vi "MarkedRobotStriker2.vi"(6 "atacando ao contrário?":bool=TRUE, 8 "Função":T1, 9 "id":u32, 10 "IA State Input":T3={"our_robots"=[], "enemy_robots"=[], "balls"=[], "geometry"={"line_width"=0, "field_length"=0, "field_width"=0, "boundary_width"=0, "referee_width"=0, "goal_width"=0, "goal_depth"=0, "goal_wall_width"=0, "center_circle_radius"=0, "defense_radius"=0, "defense_stretch"=0, "free_kick_from_defense_dist"=0, "penalty_spot_from_field_line_dist"=0, "penalty_line_from_spot_dist"=0}, "IA Judge"={"stage"="", "command"="", "our_goalie_id"=0.0, "enemy_goalie_id"=0.0, "command enum"=enum."Halt", "Time"=enum."Azul"}, "Received Timestamp"=timestamp(0 s since 1904-01-01), "Events"={"Touch"=FALSE, "Ball out"=FALSE, "id touch"=0.0, "Ball out of \nVision"=FALSE, "Ball inside \nGoalie area"=FALSE, "Robot not responding"=FALSE, "Robots responding status"=[1.0, 1.0, 1.0, 1.0, 1.0, 1.0], "Enemy Ball \nPossession"=FALSE, "Pass State"=FALSE, "id end of pass"=0.0, "Kick"=FALSE, "Id ini Possession"=0.0, "Ball Possesion"=FALSE, "Id Possesion"=0.0, "Direct Kick"=FALSE, "2nd Strk Ativo"=FALSE}}, 11 "AI Parameters":T2={"GotoKick"={"Dist do cone a frente"=150.0, "attacker farback"=1500.0, "Perto"=300.0, "min dist to kick"=150.0, "kick eps"=0.0, "Time to transition"=0.05}, "Attacker"={"CC chute"=0.09, "CC passe"=0.045, "Kick Force"=100.0, "ball-robot Kick"=200.0, "ball-robot Pass"=0.3, "drible\nAttk"=FALSE}, "Defender"={"D max"=1700.0, "Vel p/ robô av"=1000.0, "Kick Force"=100.0, "D atk-def"=0.0, "D farback"=0.0, "drible\ndef"=FALSE, "drible\ngoalie"=FALSE}, "Timeout"={"Field/v in x"=6.0, "Dist Robots"=300, "Dist up in y"=300}, "Pose Striker"={"dist"=200.0, "Numeric"=-4.0, "dist 2"=200.0, "drible\nstriker"=FALSE}, "Dist Stop"=300.0, "D ball out"=200, "D central gap "=150.0, "T pass"=0.0, "Force ++"=0.0, "range kick"=0.0, "Chute alto"=TRUE, "Marcador novo"=TRUE, "drible"=FALSE, "D drible"=300.0, "Versão Striker"=enum."3", "Defesa"=enum."ManMark", "Marcador"=enum."Marcar Segndo mais perigoso", "Receptor passe"=enum."2nd Striker", "Área"=enum."Quadrada"} {"D drible" format="%#_13g"; "D central gap" format="%#_13g"; "Dist Stop" format="%#_13g"; "Pose Striker"."Numeric" format="%#_13g"; "Defender"."Kick Force" format="%#_13g"; "Defender"."Vel p/ robô av" format="%#_13g"; "Attacker"."ball-robot Kick" format="%#_13g"; "Attacker"."Kick Force" format="%#_13g"; "Attacker"."CC passe" format="%#_13g"; "Attacker"."CC chute" format="%#_13g"; "GotoKick"."kick eps" format="%#_13g"; "GotoKick"."min dist to kick" format="%#_13g"; "GotoKick"."Perto" format="%#_13g"; "GotoKick"."attacker farback" format="%#_13g"; "GotoKick"."Dist do cone a frente" format="%#_13g"}) -> (2 "Dif. tempo\ninimigo bola":dbl, 3 "Robô marcado?":bool=TRUE, 7 "menor dist":dbl)   [LabVIEW 2017]
uses:
  Core/AI Input.ctl
  Core/AI Robot.ctl
  Functions Enum.ctl
  AttackerStates.ctl
  Path Planning/RRT/PathDests.ctl
  Path Planning/RRT/PathDest.ctl
  Core/AI Ball.ctl
  Core/Field Size.ctl
  Core/AI Judge.ctl
  Command Enum.ctl
  Util/Events/Events.ctl
  AI Parameters.ctl
  d3ae8bea-2540-4cab-b848-3da8b8f91e54.vi
  <vilib>/Array/Sort 2D Array - Pop Stack.vi
  <vilib>/Array/Sort 2D Array - Push Stack.vi
panel:
  out "id inimigo \nmenor tempo":dbl
  out "Array":dbl[][](array[numeric])
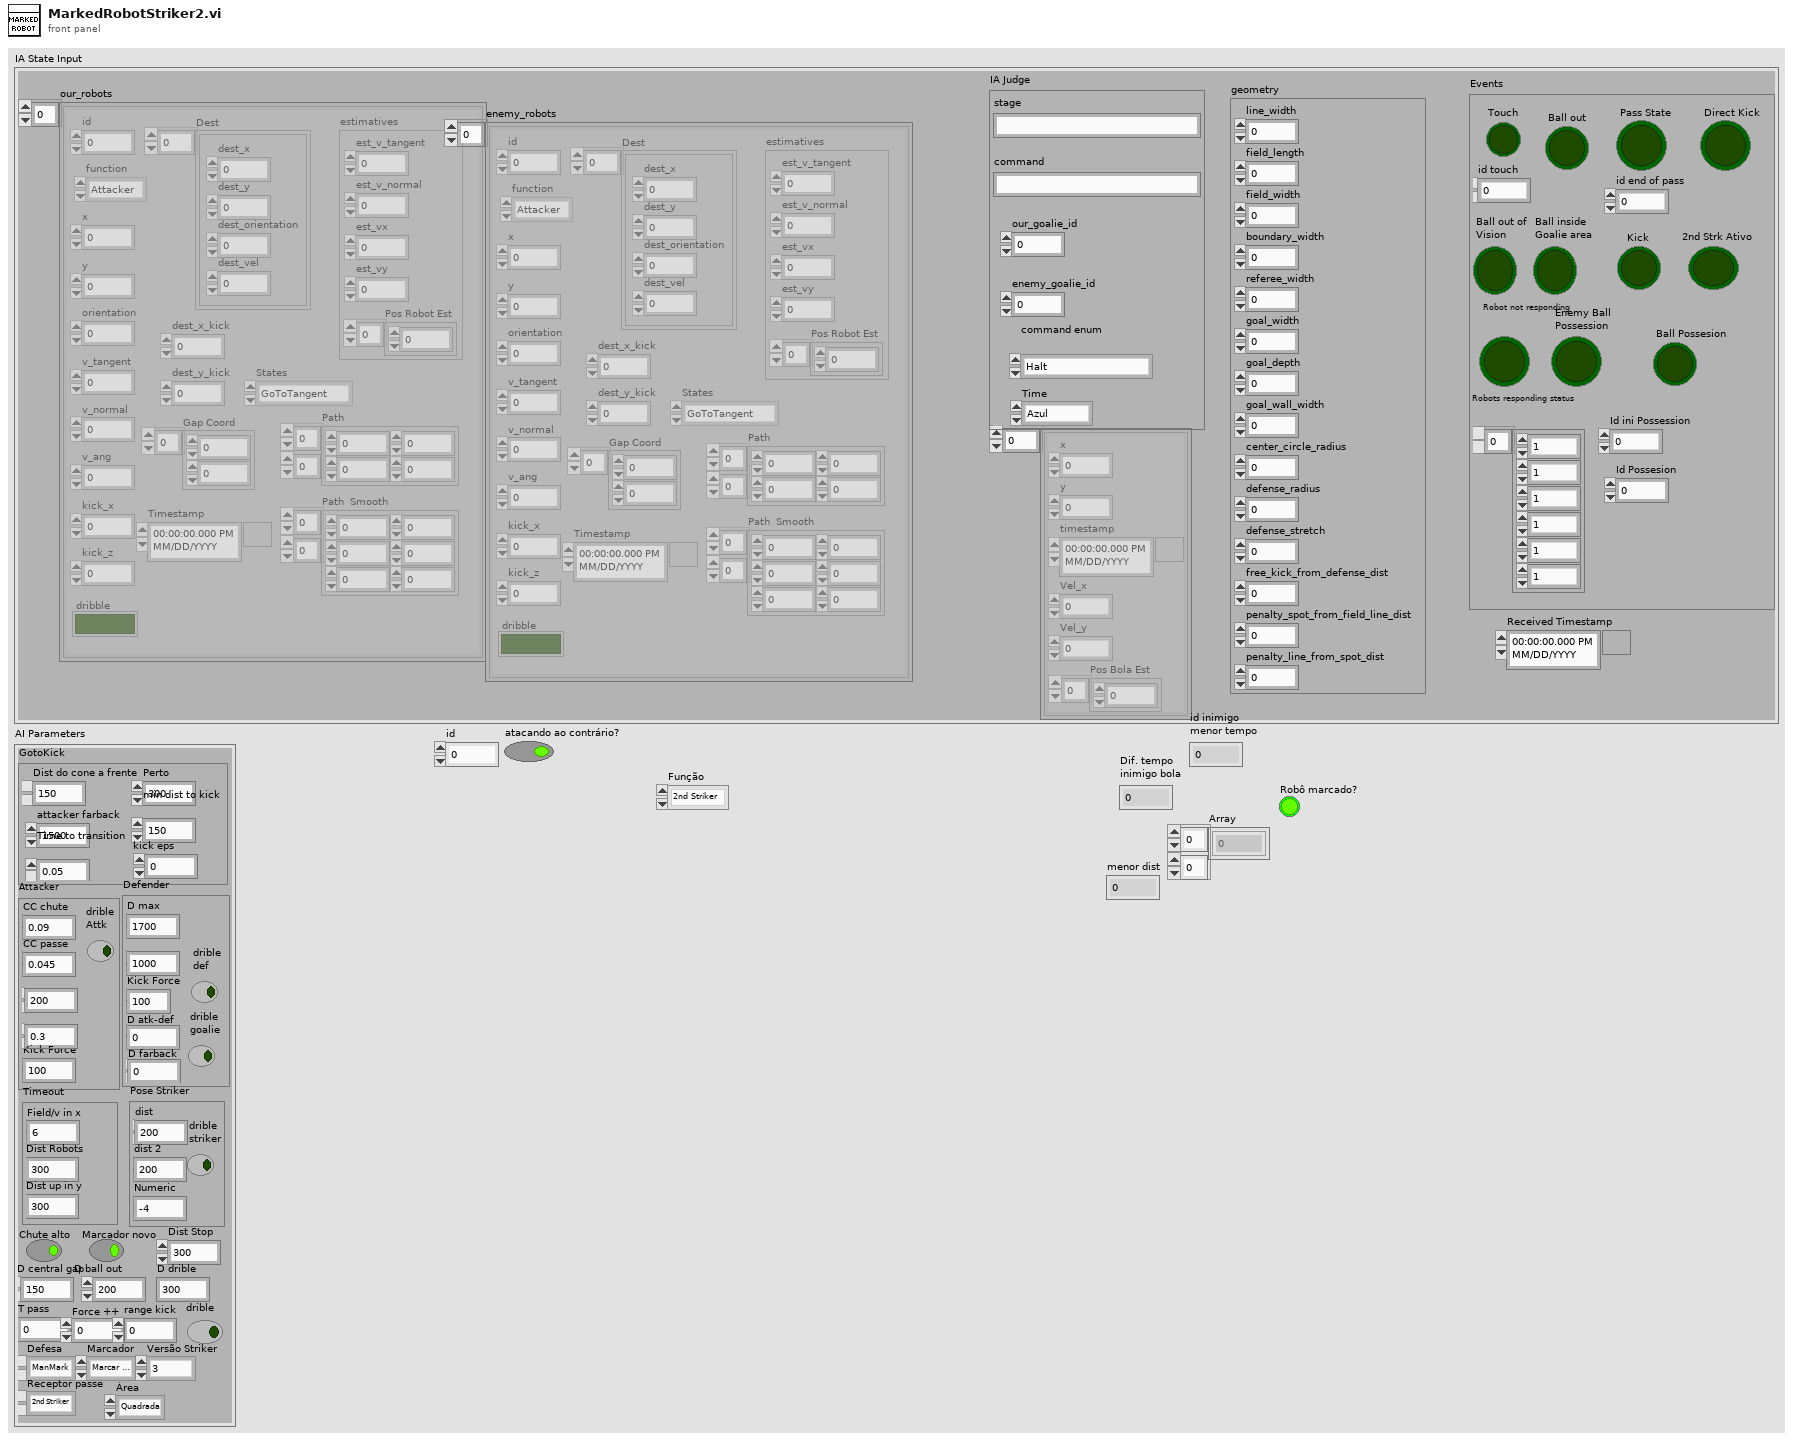
[diagram p1: front panel]
types:
  T1 = typedef "Functions Enum.ctl" = enum16{"2nd Striker", "Attacker", "Goalie", "Defender", "Striker", "Goto 0", "Dummy", "Kicker", "ZigZag 0", "ZigZag 1", "ZigZag 2", "ZigZag 3", "ZigZag 4", "ZigZag 5", "ZigZag 6", "ZigZag 7", "ZigZag 8", ""}
  T2 = typedef "AI Parameters.ctl" = cluster{"GotoKick":cluster{"Dist do cone a frente":dbl, "attacker farback":dbl, "Perto":dbl, "min dist to kick":dbl, "kick eps":dbl, "Time to transition":dbl}, "Attacker":cluster{"CC chute":dbl, "CC passe":dbl, "Kick Force":dbl, "ball-robot Kick":dbl, "ball-robot Pass":dbl, "drible\nAttk":bool}, "Defender":cluster{"D max":dbl, "Vel p/ robô av":dbl, "Kick Force":dbl, "D atk-def":dbl, "D farback":dbl, "drible\ndef":bool, "drible\ngoalie":bool}, "Timeout":cluster{"Field/v in x":dbl, "Dist Robots":u32, "Dist up in y":u32}, "Pose Striker":cluster{"dist":dbl, "Numeric":dbl, "dist 2":dbl, "drible\nstriker":bool}, "Dist Stop":dbl, "D ball out":i32, "D central gap ":dbl, "T pass":dbl, "Force ++":dbl, "range kick":dbl, "Chute alto":bool, "Marcador novo":bool, "drible":bool, "D drible":dbl, "Versão Striker":enum16{"Auto", "3", "2", "1"}, "Defesa":enum16{"ManMark", "Barreira"}, "Marcador":enum16{"Marcar Segndo mais perigoso", "Marcar o mais perigoso"}, "Receptor passe":enum16{"Auto", "2nd Striker", "Striker"}, "Área":enum16{"Quadrada", "Circular"}}
  T3 = typedef "AI Input.ctl" = cluster{"our_robots":T4[], "enemy_robots":T4[], "balls":T8[], "geometry":T9, "IA Judge":T10, "Received Timestamp":timestamp, "Events":T12}
  T4 = typedef "AI Robot.ctl" = cluster{"id":u32, "function":T1, "x":dbl, "y":dbl, "orientation":dbl, "v_tangent":dbl, "v_normal":dbl, "v_ang":dbl, "kick_x":dbl, "kick_z":dbl, "dribble":bool, "Timestamp":timestamp, "estimatives":cluster{"est_v_tangent":dbl, "est_v_normal":dbl, "est_vx":dbl, "est_vy":dbl, "Pos Robot Est":dbl[]}, "dest_x_kick":dbl, "dest_y_kick":dbl, "Gap Coord":dbl[], "States":T5, "Path ":dbl[][], "Path  Smooth":dbl[][], "Dest":T6}
  T5 = typedef "AttackerStates.ctl" = enum16{"Pass", "GoToTangent", "BallGetting", "GoToKick", ""}
  T6 = typedef "PathDests.ctl" = T7[]
  T7 = typedef "PathDest.ctl" = cluster{"dest_x":dbl, "dest_y":dbl, "dest_orientation":dbl, "dest_vel":dbl}
  T8 = typedef "AI Ball.ctl" = cluster{"x":dbl, "y":dbl, "timestamp":timestamp, "Vel_x":dbl, "Vel_y":dbl, "Pos Bola Est":dbl[]}
  T9 = typedef "Field Size.ctl" = cluster{"line_width":u32, "field_length":u32, "field_width":u32, "boundary_width":u32, "referee_width":u32, "goal_width":u32, "goal_depth":u32, "goal_wall_width":u32, "center_circle_radius":u32, "defense_radius":u32, "defense_stretch":u32, "free_kick_from_defense_dist":u32, "penalty_spot_from_field_line_dist":u32, "penalty_line_from_spot_dist":u32}
  T10 = typedef "AI Judge.ctl" = cluster{"stage":string, "command":string, "our_goalie_id":dbl, "enemy_goalie_id":dbl, "command enum":T11, "Time":enum16{"Azul", "Amarelo"}}
  T11 = typedef "Command Enum.ctl" = enum16{"Halt", "Stop", "Force Start", "PKA Normal Start", "Prepare Kickoff Ally", "PKE Normal Start", "Prepare Kickoff Enemy", "Prepare Penalty Ally", "PPA Normal Start", "Prepare Penalty Enemy", "PPE Normal Start", "Direct Free Enemy", "Direct Free Ally", "Indirect Free Enemy", "Indirect Free Ally", "Timeout Enemy", "Timeout Ally", "Goal Enemy", "Goal Ally", "Ball Placement Enemy", "Ball Placement Ally", "Normal Half Time", "Extra Time Break", "Extra Half Time", "None", "Post Game"}
  T12 = typedef "Events.ctl" = cluster{"Touch":bool, "Ball out":bool, "id touch":dbl, "Ball out of \nVision":bool, "Ball inside \nGoalie area":bool, "Robot not responding":bool, "Robots responding status":dbl[], "Enemy Ball \nPossession":bool, "Pass State":bool, "id end of pass":dbl, "Kick":bool, "Id ini Possession":dbl, "Ball Possesion":bool, "Id Possesion":dbl, "Direct Kick":bool, "2nd Strk Ativo":bool}
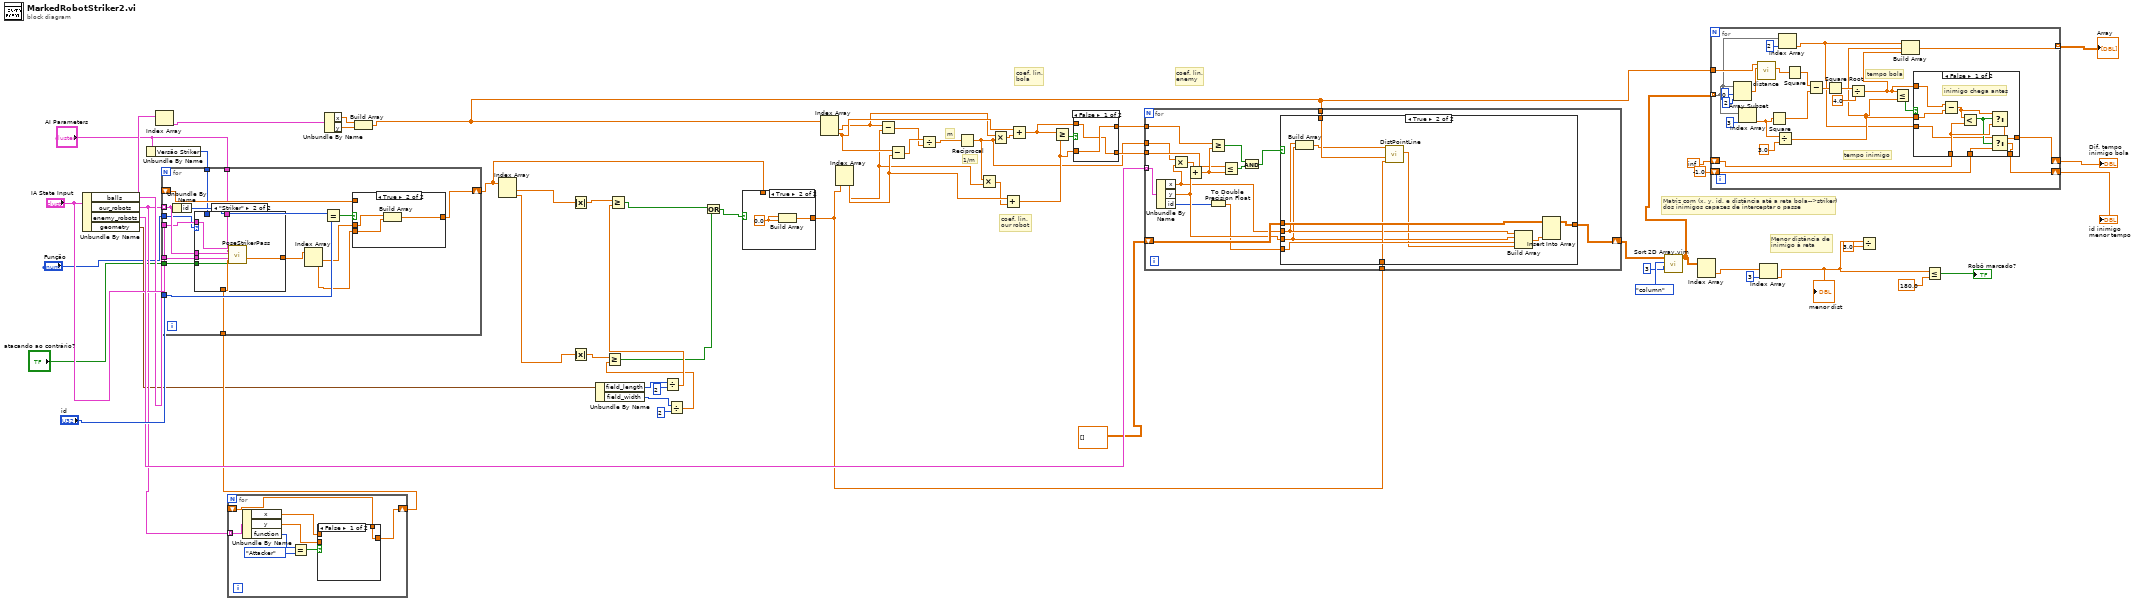
[diagram p0: block diagram]
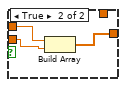
[diagram p4: hidden frame]
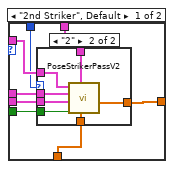
[diagram p7: hidden frame]
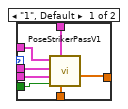
[diagram p8: hidden frame]
diagram:
  # "Menor distância de \ninimigo à reta"
  # "Matriz com (x, y, id, e distância até a reta bola-->striker) \ndos inimigos capazes de interceptar o passe"
  # "coef. lin.\nbola"
  # "coef. lin.\nenemy"
  # "coef. lin.\nour robot"
  # "1/m"
  # "m"
  n1 = Unbundle By Name("IA State Input") -> ("balls"=w38:T8[], "our_robots"=w37:T4[], "enemy_robots"=w52:T4[], "geometry"=w25:T9)
  n2 = Unbundle By Name("AI Parameters") -> ("Versão Striker"=w17:enum16{"Auto", "3", "2", "1"})
  n3 = Index Array(array=w38) -> (element=w60:T8)  [unwired: 1 in]
  n4 = for {
    tunnel: w37 -> [w69] mode=indexing
    shift-right: [w63] -> w36
    shift-left: _ -> [w62]
    n5 = Unbundle By Name(w69) -> ("x"=w65:dbl, "y"=w64:dbl, "function"=w68:T1)
    n6 = Equal?(x=w68, y=Functions_Enum."Attacker") -> (x = y?=w66:bool)
    n7 = case shown="False" w66 {
      tunnel: w65 -> [_ w73]
      tunnel: w64 -> [_ w72]
      tunnel: [w70 w71] -> w63
      tunnel: w62 -> [w70 _]
      frame False {
      }
      frame True {
        n8 = Build Array(w73, w72) -> (w71:dbl[])
      }
    }
  }
  n9 = for {
    tunnel: w37 -> [w81] mode=indexing
    tunnel: "id" -> [w88]
    shift-right: [w86] -> w20
    shift-left: _ -> [w85]
    tunnel: "IA State Input" -> [w80]
    tunnel: w38 -> [w79]
    tunnel: "AI Parameters" -> [w78]
    tunnel: w36 -> [w77]
    tunnel: "Função" -> [w76]
    tunnel: w17 -> [w75]
    tunnel: "atacando ao contrário?" -> [w74]
    n10 = Unbundle By Name(w81) -> ("id"=w89:u32)
    n11 = case shown="\"Striker\"" w76 {
      tunnel: [w97 w118] -> w84
      tunnel: w81 -> [w94 w117]
      tunnel: w80 -> [w95 w116]
      tunnel: w79 -> [w93 w115]
      tunnel: w78 -> [w96 w114]
      tunnel: w77 -> [w92 w113]
      tunnel: w75 -> [w91 _]
      tunnel: w74 -> [w90 w112]
      frame "2nd Striker", Default {
        n12 = case shown="\"2\"" w91 {
          tunnel: [w103 w111] -> w97
          tunnel: w96 -> [w100 w110]
          tunnel: w95 -> [w99 w109]
          tunnel: w94 -> [w101 w108]
          tunnel: w93 -> [w102 w107]
          tunnel: w92 -> [w104 w106]
          tunnel: w90 -> [w98 w105]
          frame "1", Default {
            n13 = call "PoseStrikerPassV1.vi"("Array"=w104, "AI Parameters"=w100, "atacando ao contrário?"=w98, "balls"=w102, "Robot in"=w101, "IA Input"=w99) -> ("FinalPosition"=w103:dbl[])  [unwired: 4 in, 1 out]
          }
          frame "2" {
            n14 = call "PoseStrikerPassV2.vi"("Array"=w106, "AI Parameters"=w110, "atacando ao contrário?"=w105, "balls"=w107, "Robot in"=w108, "IA Input"=w109) -> ("FinalPosition"=w111:dbl[])  [unwired: 4 in, 1 out]
          }
        }
      }
      frame "Striker" {
        n15 = call "PoseStrikerPass.vi"("Array"=w113, "AI Parameters"=w114, "atacando ao contrário?"=w112, "balls"=w115, "Robot in"=w117, "IA Input"=w116) -> ("FinalPosition"=w118:dbl[])  [unwired: 4 in, 1 out]
      }
    }
    n16 = Index Array(array=w84) -> (element #1=w83:dbl, element #2=w82:dbl)  [unwired: 2 in]
    n17 = Equal?(x=w89, y=w88) -> (x = y?=w87:bool)
    n18 = case shown="True" w87 {
      tunnel: w83 -> [_ w122]
      tunnel: w82 -> [_ w121]
      tunnel: [w119 w120] -> w86
      tunnel: w85 -> [w119 _]
      frame False {
      }
      frame True {
        n19 = Build Array(w122, w121) -> (w120:dbl[])
      }
    }
  }
  n20 = Unbundle By Name(w60) -> ("x"=w59:dbl, "y"=w58:dbl)
  n21 = Build Array(w59, w58) -> (w12:dbl[])
  n22 = Index Array(array=w20) -> (element #1=w24:dbl, element #2=w23:dbl)  [unwired: 2 in]
  n23 = Absolute Value(x=w24) -> (abs(x)=w31:dbl)
  n24 = Absolute Value(x=w23) -> (abs(x)=w29:dbl)
  n25 = Unbundle By Name(w25) -> ("field_length"=w35:u32, "field_width"=w32:u32)
  n26 = Divide(x=w35, y=2) -> (x/y=w30:dbl)
  n27 = Greater Or Equal?(x=w31, y=w30) -> (x >= y?=w27:bool)
  n28 = Divide(x=w32, y=u32 2) -> (x/y=w28:dbl)
  n29 = Greater Or Equal?(x=w29, y=w28) -> (x >= y?=w26:bool)
  n30 = Or(x=w27, y=w26) -> (x .or. y?=w22:bool)
  n31 = case shown="True" w22 {
    tunnel: [w123 w124] -> w21
    tunnel: w20 -> [w123 _]
    frame False {
    }
    frame True {
      w125 = 0.0
      n32 = Build Array(w125, w125) -> (w124:dbl[])
    }
  }
  n33 = Index Array(array=w12) -> (element #1=w3:dbl, element #2=w56:dbl)  [unwired: 2 in]
  n34 = Index Array(array=w21) -> (element #1=w4:dbl, element #2=w55:dbl)  [unwired: 2 in]
  n35 = Subtract(x=w3, y=w4) -> (x-y=w53:dbl)
  n36 = Subtract(x=w56, y=w55) -> (x-y=w54:dbl)
  n37 = Divide(x=w54, y=w53) -> (x/y=w57:dbl)
  n38 = Reciprocal(x=w57) -> (1/x=w1:dbl)
  n39 = Multiply(x=w1, y=w4) -> (x*y=w5:dbl)
  n40 = Multiply(x=w3, y=w1) -> (x*y=w2:dbl)
  n41 = Add(x=w55, y=w5) -> (x+y=w49:dbl)
  n42 = Add(x=w56, y=w2) -> (x+y=w50:dbl)
  n43 = Greater Or Equal?(x=w50, y=w49) -> (x >= y?=w51:bool)
  n44 = case shown="False" w51 {
    tunnel: [w127 w129] -> w48
    tunnel: w50 -> [w126 w129]
    tunnel: [w126 w128] -> w47
    tunnel: w49 -> [w127 w128]
    frame False {
    }
    frame True {
    }
  }
  n45 = for {
    tunnel: w52 -> [w146] mode=indexing
    tunnel: w1 -> [w132]
    shift-right: [w144] -> w44
    shift-left: dbl[][] [] -> [w145]
    tunnel: w48 -> [w139]
    tunnel: w47 -> [w138]
    tunnel: w12 -> [w135]
    tunnel: w21 -> [w134]
    n46 = Unbundle By Name(w146) -> ("x"=w131:dbl, "y"=w137:dbl, "id"=w133:u32)
    n47 = Multiply(x=w132, y=w131) -> (x*y=w130:dbl)
    n48 = Add(x=w130, y=w137) -> (x+y=w143:dbl)
    n49 = Greater Or Equal?(x=w139, y=w143) -> (x >= y?=w141:bool)
    n50 = To Double Precision Float(number=w133) -> (double precision float=w136:dbl)
    n51 = Less Or Equal?(x=w138, y=w143) -> (x <= y?=w142:bool)
    n52 = And(x=w141, y=w142) -> (x .and. y?=w140:bool)
    n53 = case shown="True" w140 {
      tunnel: w145 -> [w147 w157]
      tunnel: [w147 w156] -> w144
      tunnel: w131 -> [_ w151]
      tunnel: w137 -> [_ w150]
      tunnel: w136 -> [_ w155]
      tunnel: w135 -> [_ w153]
      tunnel: w134 -> [_ w152]
      frame False {
      }
      frame True {
        n54 = Build Array(w151, w150) -> (w149:dbl[])
        n55 = call "DistPointLine.vi"("P2"=w152, "P1"=w153, "Q"=w149) -> ("distance"=w148:dbl)  [unwired: 8 in]
        n56 = Build Array(w151, w150, w155, w148) -> (w154:dbl[])
        n57 = Insert Into Array(array=w157, new element=w154) -> (w156:dbl[][])  [unwired: 2 in]
      }
    }
  }
  n58 = call "Sort 2D Array.vim"("index"=3, "dimension to index (column)"=enum16{"column", "row"}."column", "2D array"=w44) -> ("sorted 2D array"=w11:dbl[][])  [unwired: 7 in, 1 out]
  n59 = Index Array(array=w11) -> (element=w13:dbl[])  [unwired: 2 in]
  n60 = for {
    tunnel: w12 -> [w162]
    tunnel: w11 -> [w161] mode=indexing
    shift-right: [w168] -> w9
    shift-left: inf -> [w167]
    tunnel: [w166] -> w8 mode=indexing
    shift-right: [w160] -> w6
    shift-left: -1.0 ("Numeric") -> [w158]
    # "tempo inimigo"
    # "tempo bola"
    n61 = Array Subset(array=w161, index=0, length=2) -> (w178:dbl[])
    n62 = Index Array(array=w161, index=3) -> (element=w171:dbl)
    n63 = call "distance.vi"("P1"=w178, "P2"=w162) -> ("Dist P1P2"=w177:dbl)  [unwired: 9 in]
    n64 = Square(x=w171) -> (x^2=w175:dbl)
    n65 = Divide(x=w171, y=3.0) -> (x/y=w164:dbl)
    n66 = Index Array(array=w161, index=2) -> (element=w159:dbl)
    n67 = Square(x=w177) -> (x^2=w176:dbl)
    n68 = Subtract(x=w176, y=w175) -> (x-y=w174:dbl)
    n69 = Square Root(x=w174) -> (sqrt(x)=w173:dbl)
    n70 = Divide(x=w173, y=4.0) -> (x/y=w165:dbl)
    n71 = Less Or Equal?(x=w165, y=w164) -> (x <= y?=w169:bool)
    n72 = Build Array(w159, w164, w165) -> (w166:dbl[])
    n73 = case shown="False" w169 {
      tunnel: w164 -> [w186 _]
      tunnel: w165 -> [w187 _]
      tunnel: [w188 w192] -> w168
      tunnel: w167 -> [w189 w192]
      tunnel: [w184 w191] -> w160
      tunnel: w159 -> [w183 _]
      tunnel: w158 -> [w182 w191]
      frame False {
        # "inimigo chega antes"
        n74 = Subtract(x=w187, y=w186) -> (x-y=w190:dbl)
        n75 = Less?(x=w190, y=w189) -> (x < y?=w185:bool)
        n76 = Select(t=w190, s=w185, f=w189) -> (s? t:f=w188:dbl)
        n77 = Select(t=w183, s=w185, f=w182) -> (s? t:f=w184:dbl)
      }
      frame True {
        # "bola passa antes"
      }
    }
  }
  "Dif. tempo\ninimigo bola" <- w9
  "Array" <- w8
  "id inimigo \nmenor tempo" <- w6
  n78 = Index Array(array=w13, index=3) -> (element=w15:dbl)
  "menor dist" <- w15
  n79 = Divide(x=w15, y=3.0) -> ()  [unwired: 1 out]
  n80 = Less Or Equal?(x=w15, y=180.0) -> (x <= y?=→"Robô marcado?":bool)
